vi "SEA-9811_ReceiverAndTransmitter_FPGA_IO_simulated.vi"() -> ()   [LabVIEW 2012]
doc: "This example demonstrates the receiver's functionality. ARINC data can be received with up to 8 channels which can be configured regarding high- or low-speed data rate, label recognition, parity check, decoder functions or label bit order (CONFIG). Up to sixteen 8-bit labels can be stored for label recognition. Duplicate values if you need fewer labels. For more details, look at the RT frontend example.\n\nCopyright (c) 2013 S.E.A. Datentechnik GmbH, Germany"
uses:
  <vilib>/Platform/TimedLoop/XDataNode/timing_clust.ctl
  <vilib>/Platform/TimedLoop/XDataNode/nitl_modes.ctl
  <vilib>/Platform/TimedLoop/XDataNode/wakeup.ctl
  <vilib>/rvi/Emulation/niFpgaSctlEmulationGetInTimedLoop.vi
  <vilib>/rvi/Emulation/niFpgaSctlEmulationGlobalWrite.vi
  <vilib>/rvi/interface/RandomDataEmulation/nirviRandomDataFPGAFIFO.vi
  <vilib>/rvi/interface/RandomDataEmulation/niFpgaRandomDataHandleErrors.vi
  <vilib>/rvi/Emulation/niFpgaSctlEmulationRegisterWithScheduler.vi
  <vilib>/rvi/Emulation/niFpgaSctlEmulationScheduler.vi
  <vilib>/Platform/TimedLoop/XDataNode/XDataNode.xnode
  <vilib>/rvi/DataTransferAndStorage/Container/XNode/niFpgaContainer.xnode
  <vilib>/rvi/interface/RandomDataEmulation/nirviRandomDataFpgaReadWriteTemplate.vi
  <vilib>/rvi/eio/common/nirviEmuTemplateMethod_errors.vi
  <vilib>/eio/EIOPropertyNode/EIOPropertyNode.xnode
  <vilib>/eio/EIOMethodNode/EIOMethodNode.xnode
  <vilib>/eio/EIONode/EIONode.xnode
  <vilib>/rvi/eio/common/nirviEmuTemplatePropertyGet_errors.vi
  <vilib>/rvi/eio/common/nirviEmuTemplatePropertyGet_noerrors.vi
  <vilib>/rvi/eio/common/nirviEmuTemplatePropertySet_errors.vi
  <vilib>/rvi/eio/common/nirviEmuTemplatePropertySet_noerrors.vi
  <userlib>/FPGA Timekeeper 1.1b0/FPGA Timekeeper.lvlib
  <vilib>/Platform/TimedLoop/XDataNode/XDNodeRunTimeDep.lvlib
panel:
  in  "Rx Label Filter":u8[](array[numeric])=[0, 0, 0, 0, 0, 0, 0, 0, 0, 0, 0, 0, 0, 0, 0, 0]
  in  "RxSimRate(us)":u32=500 caption="Count(mSec)"
  out "Rx rate us":u32
  out "Elements in FIFO":u32
  out "FPGA Timekeeper time (ns)":u64
  out "FPGA Timekeeper locked":bool
  out "offset from RT time (ns)":i32
  in  "RT time (ns)":u64
  in  "Finished config":bool
  in  "Configure\nchannel":bool
  out "Rx Status":u16 format="%016b"
  out "Tx Status":u8 format="%08b"
  in  "Tx Data":u32=305419896 format="%08x"
  in  "Tx Config Data (TCR)":u16=8192 format="%04x"
  in  "Transmit Data":bool
  out "DMA Overflow":bool
  in  "Rx Channel Number":u8 max=7 step=1
  in  "Rx Config Data (RCR)":u16=32 format="%04x"
  # "Please refer to VI description for instructions!"
  # "Receiver Configuration"
  # "DMA Status"
  # "Transmitter"
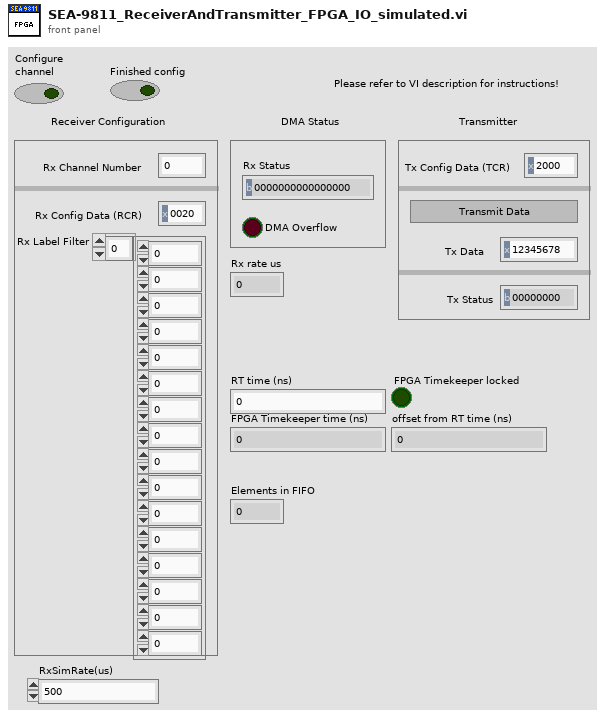
[diagram p1: front panel]
types:
  T1 = cluster{"Rx Label Filter[0]":u8, "Rx Label Filter[1]":u8, "Rx Label Filter[2]":u8, "Rx Label Filter[3]":u8, "Rx Label Filter[4]":u8, "Rx Label Filter[5]":u8, "Rx Label Filter[6]":u8, "Rx Label Filter[7]":u8, "Rx Label Filter[8]":u8, "Rx Label Filter[9]":u8, "Rx Label Filter[10]":u8, "Rx Label Filter[11]":u8, "Rx Label Filter[12]":u8, "Rx Label Filter[13]":u8, "Rx Label Filter[14]":u8, "Rx Label Filter[15]":u8}
  T2 = typedef "ARINC word.ctl" = u32
  T3 = typedef "XDNodeRunTimeDep.lvlib/timing_clust.ctl" = cluster{"Expected End [f-1]":u64, "Actual End [f-1]":u64, "Finished Late? [f-1]":bool, "Expected End [i-1]":u64, "Actual End [i-1]":u64, "Finished Late? [i-1]":bool, "Expected Start [i]":u64, "Actual Start [i]":u64, "Expected Start [f]":u64, "Actual Start [f]":u64, "Source Name":string, "Structure Name":string, "Period":i64, "Deadline":i64, "Offset":i64, "Start":i64, "Priority":i32, "Timeout":i32, "Mode":T4, "Wakeup Reason":T5, "Error":errorcluster, "Source Type":string, "Secondary Source Type":string, "Global End Time":u64, "Global Start Time":u64, "Frame Duration":u64, "Iteration Duration":u64, "Assigned CPU":i32, "I/O Scan Engine Mode":u32}
  T4 = typedef "XDNodeRunTimeDep.lvlib/nitl_modes.ctl" = enum32{"No Change", "Process missed periods, maintain original phase", "Discard missed periods, maintain original phase", "Process missed periods, ignore original phase", "Discard missed periods, ignore original phase"}
  T5 = typedef "XDNodeRunTimeDep.lvlib/wakeup.ctl" = enum32{"Normal", "Aborted", "Asynchronous wakeup", "Timing source error", "Timed loop error", "Timeout"}
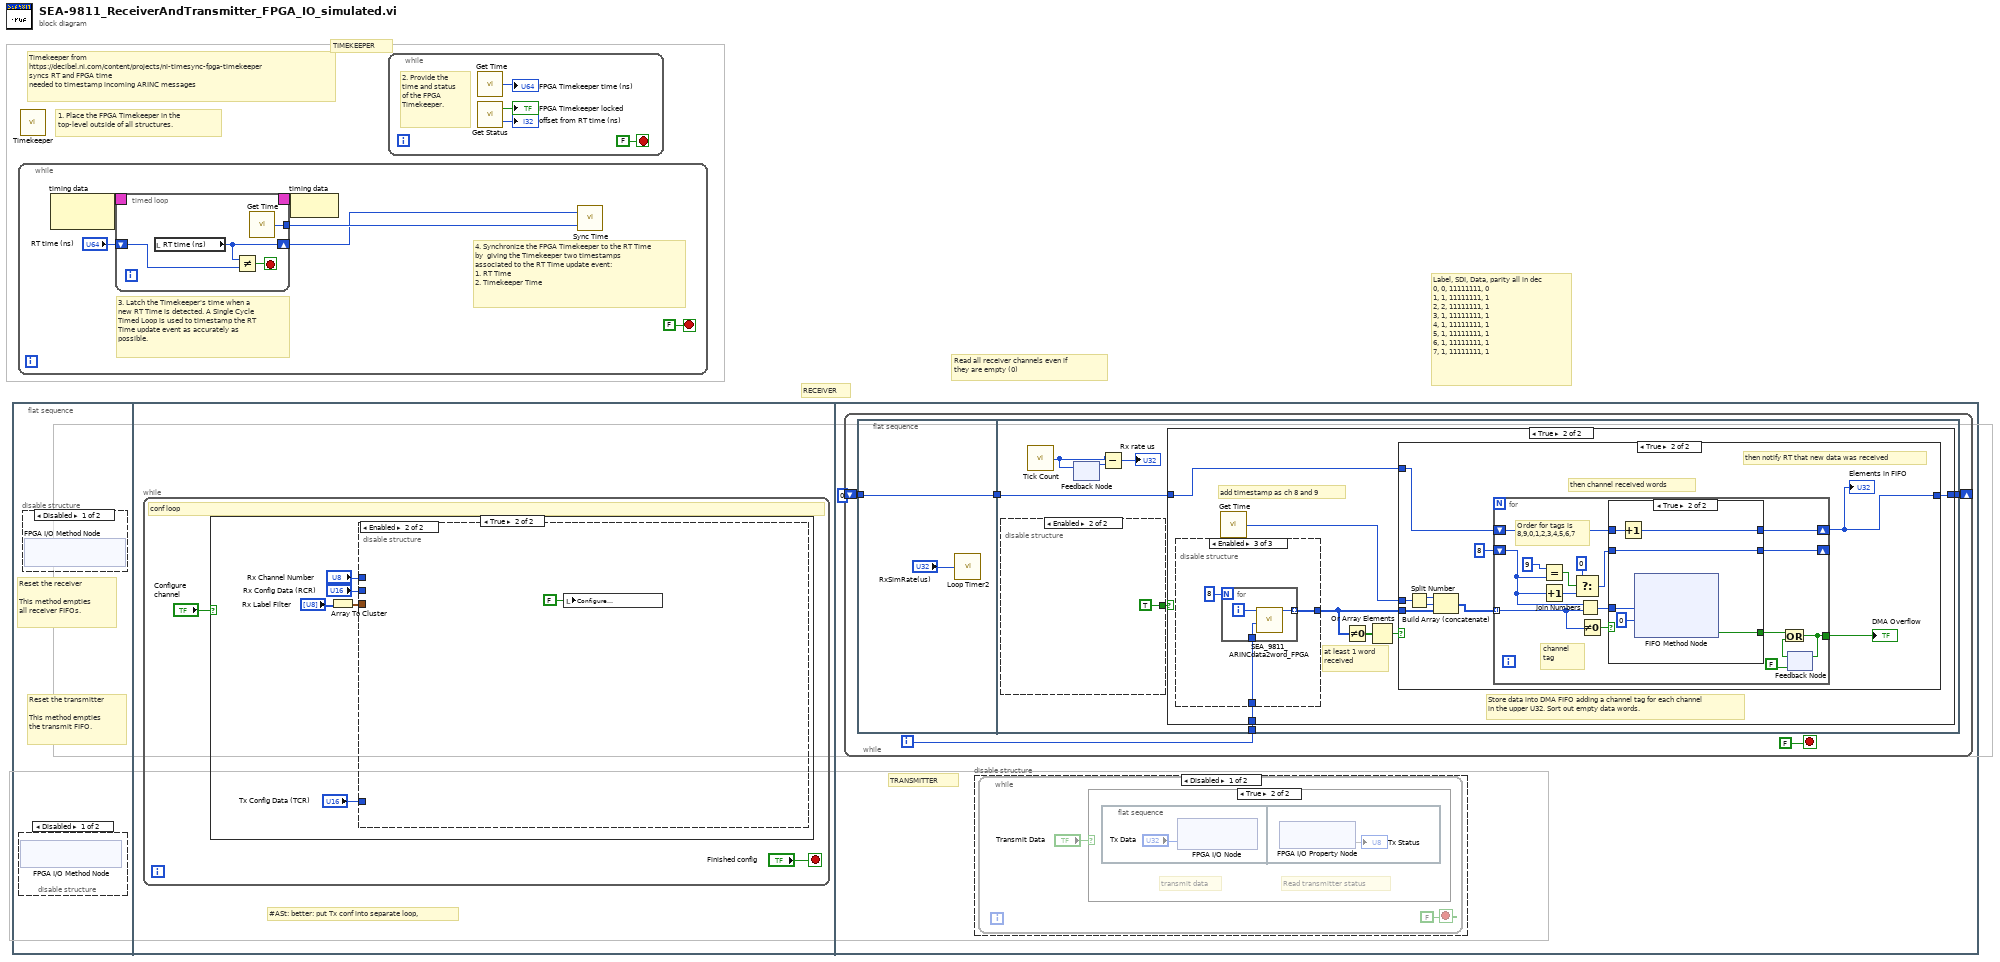
[diagram p0: block diagram]
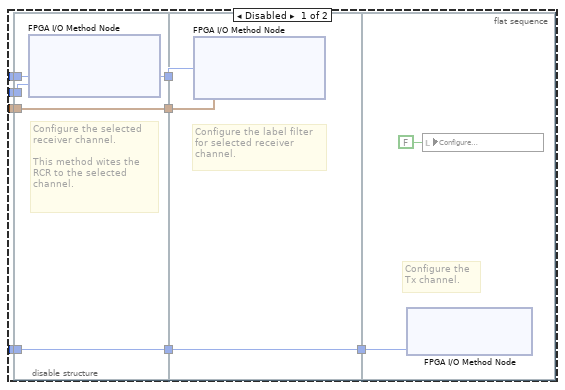
[diagram p5: hidden frame]
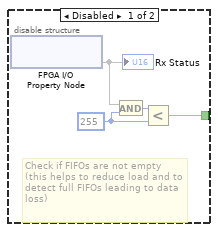
[diagram p8: hidden frame]
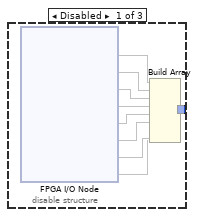
[diagram p10: hidden frame]
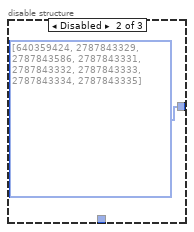
[diagram p11: hidden frame]
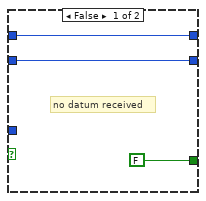
[diagram p13: hidden frame]
diagram:
  # "Label, SDI, Data, parity all in dec\n0, 0, 11111111, 0 \n1, 1, 11111111, 1 \n2, 2, 11111111, 1\n3, 1, 11111111, 1 \n4, 1, 11111111, 1 \n5, 1, 11111111, 1 \n6, 1, 11111111, 1 \n7, 1, 11111111, 1"
  # "Read all receiver channels even if they are empty (0)"
  # "TIMEKEEPER"
  # "Timekeeper from\nhttps://decibel.ni.com/content/projects/ni-timesync-fpga-timekeeper\nsyncs RT and FPGA time\nneeded to timestamp incoming ARINC messages"
  # "1. Place the FPGA Timekeeper in the top-level outside of all structures."
  # "RECEIVER"
  n1 = flat-sequence {
    frame #0 {
      # "Reset the transmitter\n\nThis method empties\nthe transmit FIFO."
      # "Reset the receiver\n\nThis method empties\nall receiver FIFOs."
      n2 = disable-structure shown="Disabled" {
        frame Disabled {
          n3 = xnode "FPGA I/O Method Node"() -> ()  [unwired: 1 in, 1 out]
        }
        frame Enabled {
        }
      }
      n4 = disable-structure shown="Disabled" {
        frame Disabled {
          n5 = xnode "FPGA I/O Method Node"() -> ()  [unwired: 1 in, 1 out]
        }
        frame Enabled {
        }
      }
    }
    frame #1 {
      # "#ASt: better: put Tx conf into separate loop,"
      n6 = while {
        stop <- "Finished config" stop-if-true
        # "conf loop"
        n7 = case shown="True" "Configure\nchannel" {
          frame False {
          }
          frame True {
            n8 = Array To Cluster(array="Rx Label Filter") -> (cluster=w3:T1)
            n9 = disable-structure shown="Enabled" {
              disable-tunnel: "Rx Channel Number" -> [w11 _]
              disable-tunnel: "Rx Config Data (RCR)" -> [w10 _]
              disable-tunnel: w3 -> [w9 _]
              disable-tunnel: "Tx Config Data (TCR)" -> [w8 _]
              frame Disabled {
                n10 = flat-sequence {
                  tunnel: w11 -> [w19]
                  tunnel: [w19] -> w15
                  tunnel: w10 -> [w18]
                  tunnel: [w17] -> w14
                  tunnel: w9 -> [w17]
                  tunnel: w8 -> [w16]
                  tunnel: [w16] -> w13
                  tunnel: w15 -> [w22]
                  tunnel: w14 -> [w21]
                  tunnel: [w20] -> w12
                  tunnel: w13 -> [w20]
                  tunnel: w12 -> [w24]
                  frame #0 {
                    # "Configure the selected\nreceiver channel.\n\nThis method wites the\nRCR to the selected\nchannel."
                    n11 = xnode "FPGA I/O Method Node"("Channel Number"=w19, "Control Register"=w18) -> ()  [unwired: 1 in, 1 out]
                  }
                  frame #1 {
                    # "Configure the label filter\nfor selected receiver\nchannel."
                    n12 = xnode "FPGA I/O Method Node"("Channel Number"=w22, "Label Filter"=w21) -> ()  [unwired: 1 in, 1 out]
                  }
                  frame #2 {
                    # "Configure the\nTx channel."
                    n13 = xnode "FPGA I/O Method Node"("Control Register"=w24) -> ()  [unwired: 1 in, 1 out]
                    n14 = local write "Configure\nchannel"(FALSE ("Configure\nchannel")) -> ()
                  }
                }
              }
              frame Enabled {
                n15 = local write "Configure\nchannel"(FALSE ("Configure\nchannel")) -> ()
              }
            }
          }
        }
      }
    }
    frame #2 {
      # "TRANSMITTER"
      n16 = while {
        shift-right: [w33] -> _
        shift-left: u32 0 -> [w34]
        i -> [w31]
        stop <- FALSE stop-if-true
        n17 = flat-sequence {
          tunnel: w34 -> [w37]
          tunnel: [w37] -> w32
          tunnel: [w42] -> w33
          tunnel: w32 -> [w43]
          tunnel: w31 -> [w38]
          frame #0 {
            n18 = call "Loop Timer2"("Count(uSec)"="RxSimRate(us)") -> ()  [unwired: 1 out]
          }
          frame #1 {
            n19 = disable-structure shown="Enabled" {
              disable-tunnel: [w45 TRUE] -> w44
              frame Disabled {
                w46 = u16 255 ("y")
                # "Check if FIFOs are not empty\n(this helps to reduce load and to detect full FIFOs leading to data loss)"
                n20 = xnode "FPGA I/O Property Node"() -> ("Rx Status"=w48)  [unwired: 1 in, 1 out]
                "Rx Status" <- w48
                n21 = And(x=w48, y=w46) -> (x .and. y?=w47:u16)
                n22 = Less?(x=w47, y=w46) -> (x < y?=w45:bool)
              }
              frame Enabled {
              }
            }
            n23 = call "Tick Count"() -> ("Tick Count(uSec)"=w39:u32)
            n24 = feedback #1() -> (w40:u32)  [unwired: 1 in]
            n25 = feedback-in #1(w39) -> ()
            n26 = Subtract(x=w39, y=w40) -> (x-y=→"Rx rate us":u32)
            n27 = case shown="True" w44 {
              tunnel: w43 -> [w50 w57]
              tunnel: [w50 w56] -> w42
              tunnel: w38 -> [_ w52]
              frame False {
              }
              frame True {
                # "add timestamp as ch 8 and 9"
                # "at least 1 word\nreceived"
                # "Store data into DMA FIFO adding a channel tag for each channel in the upper U32. Sort out empty data words."
                n28 = disable-structure shown="Enabled" {
                  disable-tunnel: w52 -> [_ _ w69]
                  disable-tunnel: [_ u32[] [640359424, 2787843329, 2787843586, 2787843331, 2787843332, 2787843333, 2787843334, 2787843335] w67] -> w51
                  frame Disabled {
                    n29 = xnode "FPGA I/O Node"() -> ("Mod1/Rx0"=w59, "Mod1/Rx1"=w60, "Mod1/Rx2"=w61, "Mod1/Rx3"=w62, "Mod1/Rx4"=w63, "Mod1/Rx5"=w64, "Mod1/Rx6"=w65, "Mod1/Rx7"=w58)  [unwired: 8 in, 8 out]
                    n30 = Build Array(w59, w60, w61, w62, w63, w64, w65, w58) -> ()  [unwired: 1 out]
                  }
                  frame Disabled {
                  }
                  frame Enabled {
                    n31 = for {
                      N: 8 -> [_]
                      tunnel: w69 -> [w71]
                      tunnel: [w70] -> w67 mode=indexing
                      i -> [w72]
                      n32 = call "SEA_9811_ARINCdata2word_FPGA.vi"("Data"=w71, "Label"=w72) -> ("ARINC word out"=w70:T2)  [unwired: 9 in]
                    }
                  }
                }
                n33 = call <userlib>:"Get Time.vi"() -> ("time (ns)"=w53:u64)
                n34 = Not Equal To 0?(x=w51) -> (x != 0?=w55:bool[])
                n35 = Or Array Elements(Boolean array=w55) -> (logical OR=w54:bool)
                n36 = case shown="True" w54 {
                  tunnel: w57 -> [w73 w74]
                  tunnel: [w73 w82] -> w56
                  tunnel: w51 -> [_ w79]
                  tunnel: w53 -> [_ w75]
                  frame False {
                  }
                  frame True {
                    # "then notify RT that new data was received"
                    # "then channel received words"
                    n37 = Split Number(x=w75) -> (hi(x)=w77:u32, lo(x)=w76:u32)
                    n38 = Build Array (concatenate)(w77, w76, w79) -> (w78:T2[])
                    n39 = for {
                      tunnel: w78 -> [w90] mode=indexing
                      tunnel: [w95] -> w81
                      shift-right: [w91] -> w82
                      shift-left: w74 -> [w92]
                      shift-right: [w83] -> _
                      shift-left: u32 8 ("hi") -> [w87]
                      # "Order for tags is\n8,9,0,1,2,3,4,5,6,7"
                      # "channel\ntag"
                      n40 = Equal?(x=u32 9, y=w87) -> (x = y?=w88:bool)
                      n41 = Increment(x=w87) -> (x+1=w89:u32)
                      n42 = Select(t=u32 0, s=w88, f=w89) -> (s? t:f=w84:u32)
                      n43 = Join Numbers(hi=w87, lo=w90) -> ((hi.lo)=w93:u64)
                      n44 = Not Equal To 0?(x=w90) -> (x != 0?=w94:bool)
                      n45 = case shown="True" w94 {
                        tunnel: [FALSE ("Timed Out?") w107] -> w96
                        tunnel: w93 -> [_ w104]
                        tunnel: w92 -> [w100 w106]
                        tunnel: [w100 w105] -> w91
                        tunnel: w84 -> [w99 w102]
                        tunnel: [w99 w102] -> w83
                        frame False {
                          # "no datum received"
                        }
                        frame True {
                          n46 = Increment(x=w106) -> (x+1=w105:u32)
                          n47 = xnode ("FIFO Method Node")("Element"=w104, "Timeout"=0) -> ("Timed Out?"=w107:bool)  [unwired: 1 in, 1 out]
                        }
                      }
                      n48 = feedback #2(FALSE) -> (w97:bool)
                      n49 = Or(x=w96, y=w97) -> (x .or. y?=w95:bool)
                      n50 = feedback-in #2(w95) -> ()
                    }
                    "DMA Overflow" <- w81
                    "Elements in FIFO" <- w82
                  }
                }
              }
            }
          }
        }
      }
      n51 = disable-structure shown="Disabled" {
        frame Disabled {
          n52 = while {
            stop <- FALSE stop-if-true
            n53 = case shown="True" "Transmit Data" {
              frame False {
              }
              frame True {
                # "Read transmitter status"
                # "transmit data"
                n54 = flat-sequence {
                  frame #0 {
                    n55 = xnode "FPGA I/O Node"("Mod1/Tx0"="Tx Data") -> ()  [unwired: 1 in, 1 out]
                  }
                  frame #1 {
                    n56 = xnode "FPGA I/O Property Node"() -> ("Tx Status"=→"Tx Status")  [unwired: 1 in, 1 out]
                  }
                }
              }
            }
          }
        }
        frame Enabled {
        }
      }
    }
  }
  n57 = while {
    stop <- FALSE stop-if-true
    # "3. Latch the Timekeeper's time when a new RT Time is detected. A Single Cycle Timed Loop is used to timestamp the RT Time update event as accurately as possible."
    # "4. Synchronize the FPGA Timekeeper to the RT Time by  giving the Timekeeper two timestamps associated to the RT Time update event:\n1. RT Time\n2. Timekeeper Time"
    n58 = node-c288() -> (w113:T3)  [unwired: 1 in]
    n59 = timed-loop {
      timing: w113 -> [_]
      timing-out: [_] -> w112
      shift-right: [w114] -> w108
      shift-left: "RT time (ns)" -> [w115]
      tunnel: [w117] -> w111
      stop <- w116 stop-if-true
      n60 = local read "RT time (ns)"() -> (w114:u64)
      n61 = Not Equal?(x=w114, y=w115) -> (x != y?=w116:bool)
      n62 = call <userlib>:"Get Time.vi"() -> ("time (ns)"=w117:u64)
    }
    n63 = node-c288(w112) -> ()
    n64 = call <userlib>:"Sync Time.vi"("FPGA Timekeeper time (ns)"=w111, "time reference time (ns)"=w108) -> ()
  }
  n65 = call <userlib>:"Timekeeper.vi"() -> ()  [unwired: 12 in]
  n66 = while {
    stop <- FALSE stop-if-true
    # "2. Provide the time and status of the FPGA Timekeeper."
    n67 = call <userlib>:"Get Time.vi"() -> ("time (ns)"=→"FPGA Timekeeper time (ns)":u64)
    n68 = call <userlib>:"Get Status.vi"() -> ("FPGA Timekeeper locked"=→"FPGA Timekeeper locked":bool, "offset from time reference"=→"offset from RT time (ns)":i32)
  }
